vi "Scan Driver (for Setup UI).vi"(8 "error in (no error)":errorcluster, 11 "Scan Driver.lvclass in":refnum<class "Scan Driver.lvclass">) -> (0 "error out":errorcluster, 3 "Scan Driver.lvclass out":refnum<class "Scan Driver.lvclass">)   [LabVIEW 2017, in "Scan Driver.lvclass"]
doc: "Constructor. Finish construction of the Scan Driver after running the Setup UI methods on its component classes."
uses:
  Scan Driver.lvclass
  File IO/File IO.lvclass
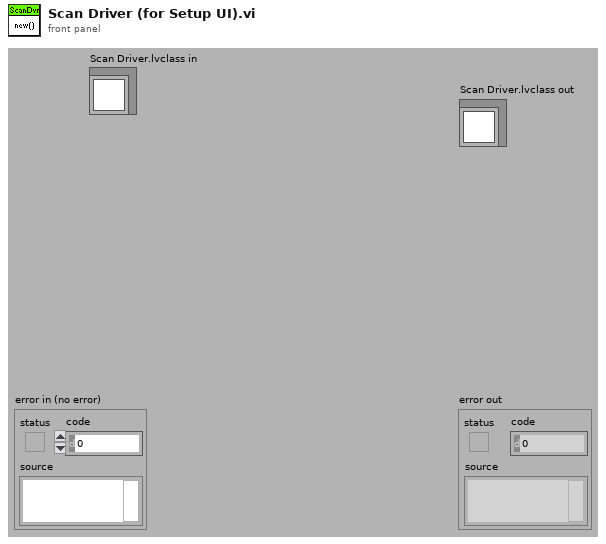
[diagram p1: front panel]
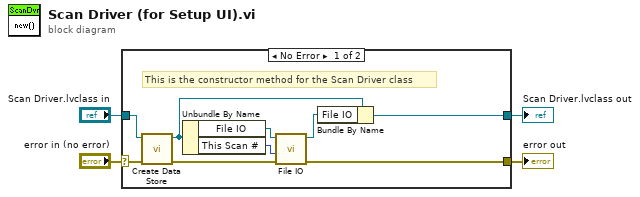
[diagram p0: block diagram]
diagram:
  n1 = case shown="No Error" "error in (no error)" {
    selector: "error in (no error)" -> [w13 w14]
    tunnel: [w10 w14] -> w3
    tunnel: [w5 w15] -> w1
    tunnel: "Scan Driver.lvclass in" -> [w12 w15]
    frame No Error {
      # "This is the constructor method for the Scan Driver class"
      n2 = call "Create Data Store.vi"("error in (no error)"=w13, "Scan Driver.lvclass in"=w12) -> ("error out"=w11:errorcluster, "Scan Driver.lvclass out"=w8:refnum<class "Scan Driver.lvclass">)  [unwired: 8 out]
      n3 = Unbundle By Name(w8) -> ("File IO"=w9:refnum<class "File IO.lvclass">, "This Scan #"=w6:u32)
      n4 = call "File IO.vi"("error in"=w11, "This Scan #"=w6, "File IO in"=w9) -> ("error out"=w10:errorcluster, "File IO out"=w7:refnum<class "File IO.lvclass">)  [unwired: 7 out]
      n5 = Bundle By Name(cluster=w8, "File IO"=w7) -> (w5:refnum<class "Scan Driver.lvclass">)
    }
    frame Error {
    }
  }
  "error out" <- w3
  "Scan Driver.lvclass out" <- w1
